vi "Check for CAN Error Message.vi"(11 "data":T1[](array[typedef]) {"payload" format="%x"; "timestamp" format="%<%.7X\n%x>T"; "type" items=["CAN Data"=0, "CAN Remote"=1, "CAN Bus Error"=2, "CAN 2.0 Data"=8, "CAN FD Data"=16, "CAN FD+BRS Data"=24, "J1939 Data"=192, "Delay"=224, "Log Trigger"=225, "Start Trigger"=226]; "identifier" format="%x"}) -> (2 "Error Number":u8, 3 "Error":bool)   [LabVIEW 2025]
uses:
  <vilib>/xnet/xnet.llb/XNET Frame CAN.ctl
  <vilib>/xnet/xnet.llb/XNET Frame Type CAN.ctl
panel:
  in  "ID ERROR MESSAGE":u32=255 format="%x"
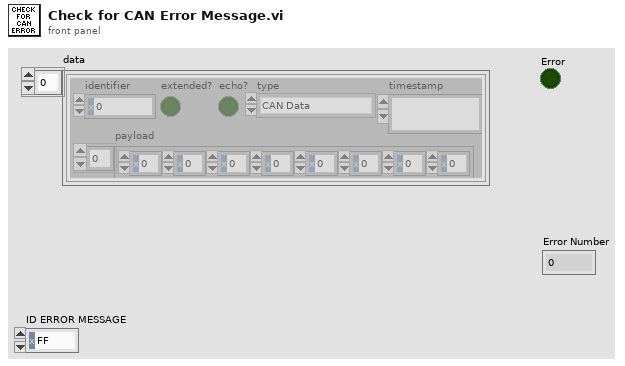
[diagram p1: front panel]
types:
  T1 = typedef "XNET Frame CAN.ctl" = cluster{"timestamp":timestamp, "payload":u8[], "identifier":u32, "type":T2, "extended?":bool, "echo?":bool}
  T2 = typedef "XNET Frame Type CAN.ctl" = u8
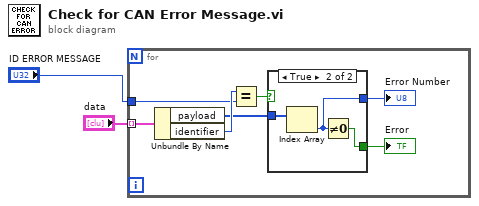
[diagram p0: block diagram]
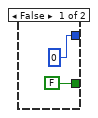
[diagram p2: hidden frame]
diagram:
  n1 = for {
    tunnel: "data" -> [w6] mode=indexing
    tunnel: "ID ERROR MESSAGE" -> [w4]
    n2 = Unbundle By Name(w6) -> ("payload"=w3:u8[], "identifier"=w5:u32)
    n3 = Equal?(x=w5, y=w4) -> (x = y?=w9:bool)
    n4 = case shown="True" w9 {
      tunnel: w3 -> [_ w14]
      tunnel: [FALSE w13] -> w8
      tunnel: [u8 0 ("Numeric") w12] -> w7
      frame False {
      }
      frame True {
        n5 = Index Array(array=w14) -> (element=w12:u8)  [unwired: 1 in]
        n6 = Not Equal To 0?(x=w12) -> (x != 0?=w13:bool)
      }
    }
    "Error" <- w8
    "Error Number" <- w7
  }
